vi "checkFinishNormalDefensivePlay.vi"(8 "error in (no error)":errorcluster, 10 "Game":refnum<class "Game.lvclass">, 11 "NormalDefensivePlay in":refnum<class "NormalDefensivePlay.lvclass">) -> (0 "error out":errorcluster, 2 "Boolean":bool, 3 "NormalDefensivePlay out":refnum<class "NormalDefensivePlay.lvclass">)   [LabVIEW 2023, in "NormalDefensivePlay.lvclass"]
uses:
  NormalDefensivePlay.lvclass
  Game_class/Game.lvclass
  NormalDefensiveWithDuelistPlay_class/NormalDefensiveWithDuelistPlay.lvclass
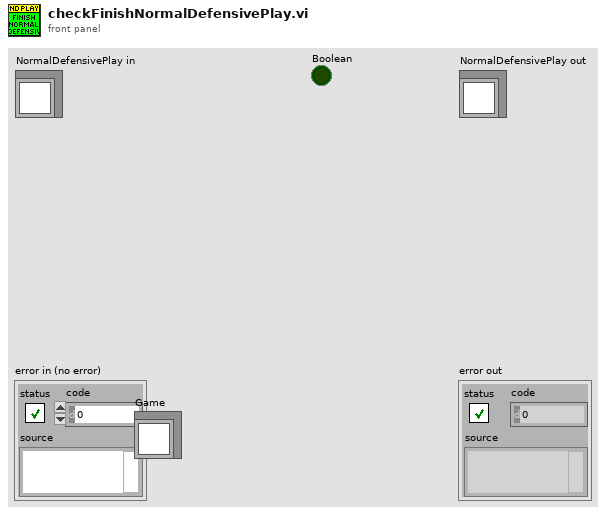
[diagram p1: front panel]
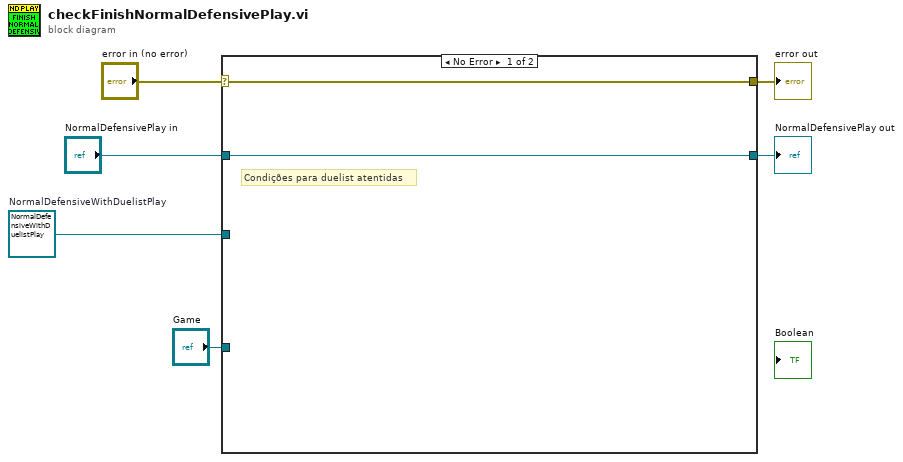
[diagram p0: block diagram]
diagram:
  w1 = refnum<class "NormalDefensiveWithDuelistPlay.lvclass"> refnum  # NormalDefensiveWithDuelistPlay
  n1 = case shown="No Error" "error in (no error)" {
    selector: "error in (no error)" -> [w7 w10]
    tunnel: [w7 w10] -> w5
    tunnel: [w8 w9] -> w3
    tunnel: "NormalDefensivePlay in" -> [w8 w9]
    tunnel: "Game" -> [_ _]
    tunnel: w1 -> [_ _]
    frame No Error {
      # "Condições para duelist atentidas"
    }
    frame Error {
    }
  }
  "error out" <- w5
  "NormalDefensivePlay out" <- w3
